vi "FilterDynamixelPositions.vi"(8 "Queue timeout (ms)":i32=8, 10 "DynamixelPosition Queue":refnum<queue>, 11 "NotifierReff":T1) -> ()   [LabVIEW 2013]
doc: "Performs and filtering that we want (default is no filtering) and writes the data to the notifier. If no data is in the queue this VI times out after 'Queue timeout (ms)' has passed and nothing is written to the notifier. When only one Dynamixel times, then '-1' is written to the timed out Dynamixel and the other torque is written to the notifier.\n\nEric Schneider, March 2014"
uses:
  Data/TypeDefs/Notifiers.ctl
  Data/TypeDefs/UTM Location.ctl
  Data/TypeDefs/Sail Set Suggestions.ctl
  Data/TypeDefs/Rudder Set Suggestions.ctl
  Data/TypeDefs/OverrideInformation.ctl
  Data/TypeDefs/OverrideMode.ctl
  Data/TypeDefs/MotorSetup.ctl
  Data/TypeDefs/DynamixelSetupInfo.ctl
  Data/TypeDefs/AirmarStatus.ctl
  Data/TypeDefs/HardwareOnline.ctl
panel:
  out "Old Rudder position":dbl
  out "New Rudder position":dbl
  out "New Jib position":dbl
  out "Old Jib position":dbl
  out "Old Main position":dbl
  out "New Main position":dbl
  out "Change for Rudder":i32
  out "Change for Jib":i32
  out "Change for Main":i32
  # "For Debugging"
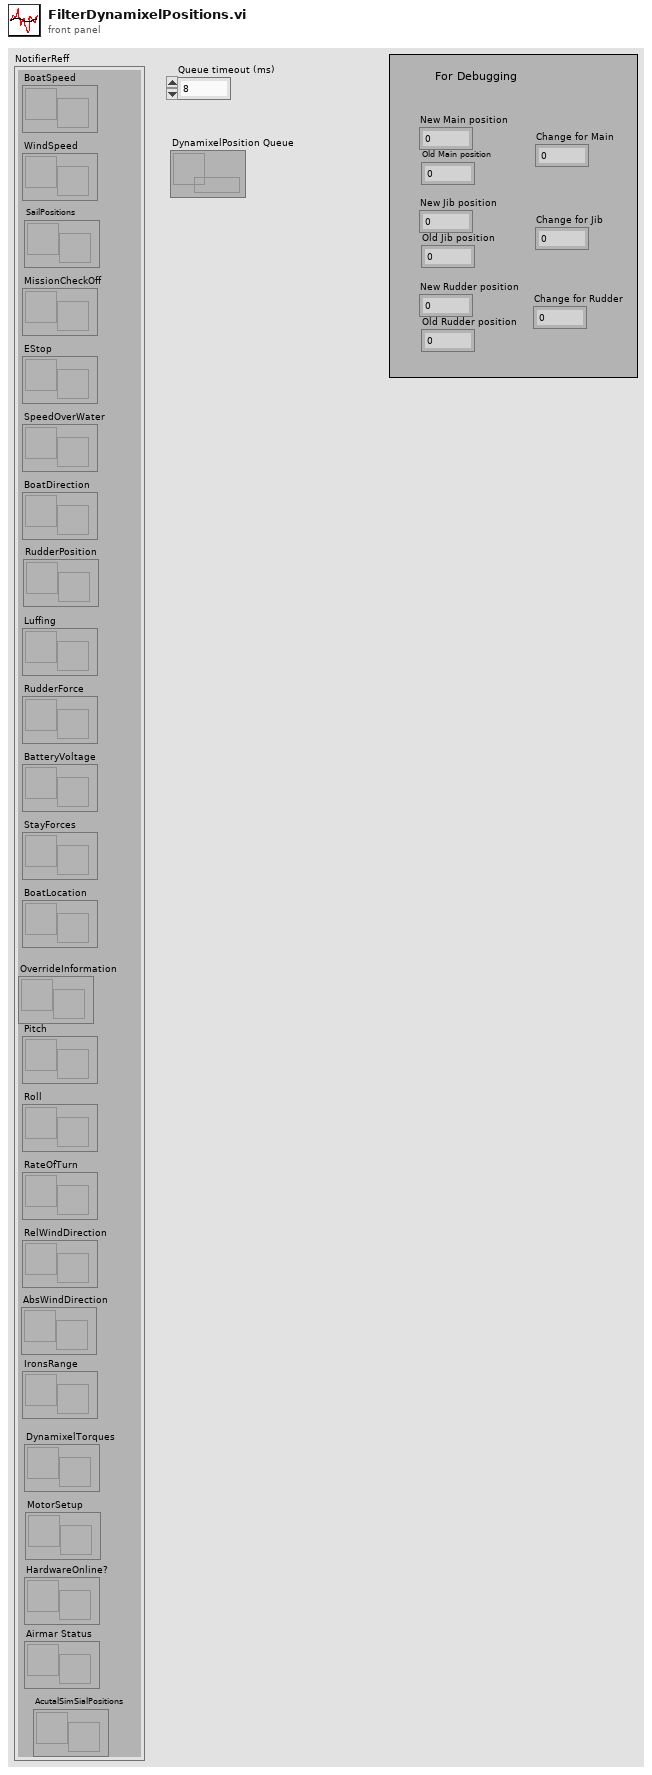
[diagram p1: front panel]
types:
  T1 = typedef "Notifiers.ctl" = cluster{"BoatSpeed":refnum<notifier>, "WindSpeed":refnum<notifier>, "MissionCheckOff":refnum<notifier>, "EStop":refnum<notifier>, "SpeedOverWater":refnum<notifier>, "BoatDirection":refnum<notifier>, "Luffing":refnum<notifier>, "RudderForce":refnum<notifier>, "BatteryVoltage":refnum<notifier>, "StayForces":refnum<notifier>, "BoatLocation":refnum<notifier>, "Pitch":refnum<notifier>, "Roll":refnum<notifier>, "RateOfTurn":refnum<notifier>, "RelWindDirection":refnum<notifier>, "SailPositions":refnum<notifier>, "RudderPosition":refnum<notifier>, "IronsRange":refnum<notifier>, "AbsWindDirection":refnum<notifier>, "OverrideInformation":refnum<notifier>, "DynamixelTorques":refnum<notifier>, "MotorSetup":refnum<notifier>, "Airmar Status":refnum<notifier>, "HardwareOnline?":refnum<notifier>, "AcutalSimSialPositions":refnum<notifier>}
  T2 = typedef "MotorSetup.ctl" = cluster{"Main Dynamixel Set Data":T3, "Rudder Dynamixel Set Data":T3, "Jib Dynamixel Set Data":T3}
  T3 = typedef "DynamixelSetupInfo.ctl" = cluster{"Lower Winch Bound":dbl, "Upper Winch Bound":dbl, "Reverse Winch Direction?":bool, "Dynamixel Cycle Number":i32}
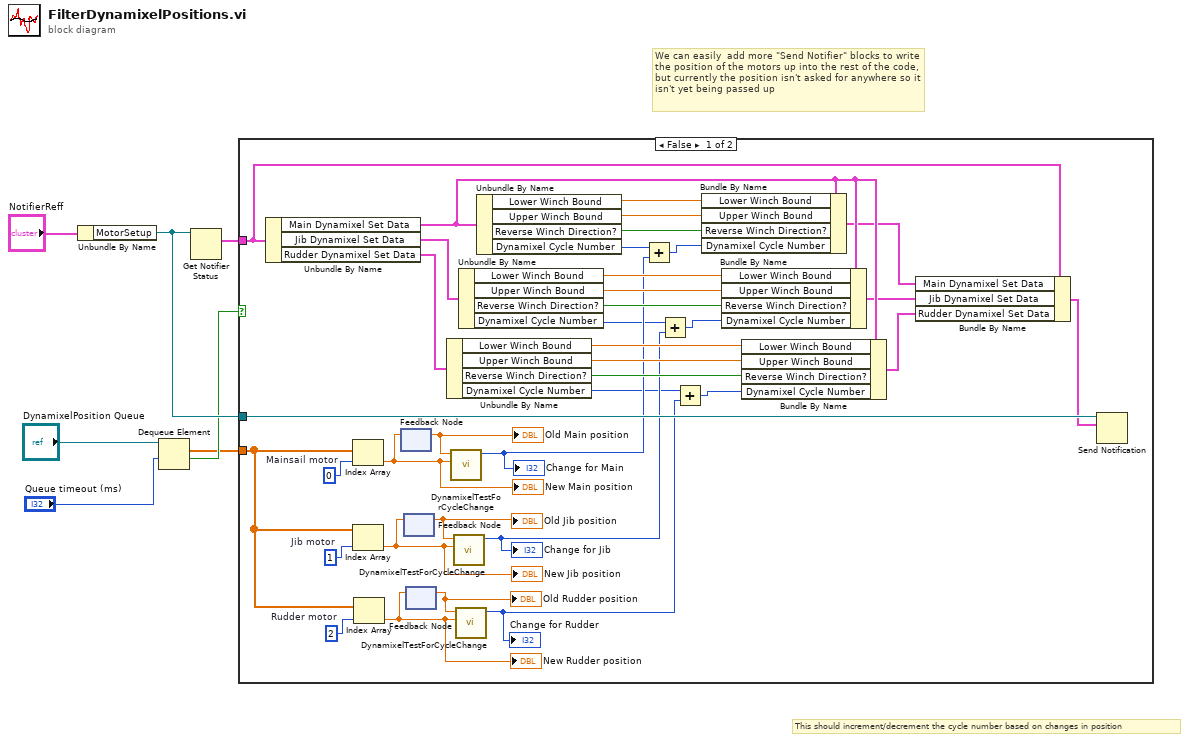
[diagram p0: block diagram]
diagram:
  # "We can easily  add more \"Send Notifier\" blocks to write the position of the motors up into the rest of the code, but currently the position isn't asked for anywhere so it isn't yet being passed up"
  # "This should increment/decrement the cycle number based on changes in position"
  n1 = Unbundle By Name("NotifierReff") -> ("MotorSetup"=w4:refnum<notifier>)
  n2 = Dequeue Element(queue="DynamixelPosition Queue", timeout in ms (-1)="Queue timeout (ms)") -> (element=w1:dbl[], timed out?=w2:bool)  [unwired: 1 in, 2 out]
  n3 = Get Notifier Status(notifier=w4) -> (current notification=w3:T2)  [unwired: 1 in, 4 out]
  n4 = case shown="False" w2 {
    tunnel: w4 -> [w42 _]
    tunnel: w3 -> [w37 _]
    tunnel: w1 -> [w23 _]
    frame False {
      w24 = 0  # Mainsail motor
      w25 = 1  # Jib motor
      w26 = 2  # Rudder motor
      n5 = Unbundle By Name(w37) -> ("Main Dynamixel Set Data"=w38:T3, "Jib Dynamixel Set Data"=w44:T3, "Rudder Dynamixel Set Data"=w43:T3)
      n6 = Index Array(array=w23, index=w24) -> (element=w22:dbl)
      "New Main position" <- w22
      n7 = Index Array(array=w23, index=w25) -> (element=w19:dbl)
      "New Jib position" <- w19
      n8 = Index Array(array=w23, index=w26) -> (element=w17:dbl)
      "New Rudder position" <- w17
      n9 = feedback #1() -> (w21:dbl)  [unwired: 1 in]
      "Old Main position" <- w21
      n10 = feedback-in #1(w22) -> ()
      n11 = feedback #2() -> (w20:dbl)  [unwired: 1 in]
      "Old Jib position" <- w20
      n12 = feedback-in #2(w19) -> ()
      n13 = feedback #3() -> (w18:dbl)  [unwired: 1 in]
      "Old Rudder position" <- w18
      n14 = feedback-in #3(w17) -> ()
      n15 = Unbundle By Name(w43) -> ("Lower Winch Bound"=w30:dbl, "Upper Winch Bound"=w29:dbl, "Reverse Winch Direction?"=w28:bool, "Dynamixel Cycle Number"=w10:i32)
      n16 = call "DynamixelTestForCycleChange.vi"("New position (deg)"=w22, "Old position (deg)"=w21) -> ("Dynamixel Cycle Number"=w15:i32)  [unwired: 9 in]
      "Change for Main" <- w15
      n17 = call "DynamixelTestForCycleChange.vi"("New position (deg)"=w19, "Old position (deg)"=w20) -> ("Dynamixel Cycle Number"=w12:i32)  [unwired: 9 in]
      "Change for Jib" <- w12
      n18 = call "DynamixelTestForCycleChange.vi"("New position (deg)"=w17, "Old position (deg)"=w18) -> ("Dynamixel Cycle Number"=w8:i32)  [unwired: 9 in]
      "Change for Rudder" <- w8
      n19 = Unbundle By Name(w44) -> ("Lower Winch Bound"=w33:dbl, "Upper Winch Bound"=w32:dbl, "Reverse Winch Direction?"=w31:bool, "Dynamixel Cycle Number"=w13:i32)
      n20 = Unbundle By Name(w38) -> ("Lower Winch Bound"=w39:dbl, "Upper Winch Bound"=w40:dbl, "Reverse Winch Direction?"=w41:bool, "Dynamixel Cycle Number"=w16:i32)
      n21 = Add(x=w16, y=w15) -> (x+y=w14:i32)
      n22 = Add(x=w13, y=w12) -> (x+y=w11:i32)
      n23 = Add(x=w10, y=w8) -> (x+y=w9:i32)
      n24 = Bundle By Name(cluster=w38, "Lower Winch Bound"=w39, "Upper Winch Bound"=w40, "Reverse Winch Direction?"=w41, "Dynamixel Cycle Number"=w14) -> (w36:T3)
      n25 = Bundle By Name(cluster=w38, "Lower Winch Bound"=w33, "Upper Winch Bound"=w32, "Reverse Winch Direction?"=w31, "Dynamixel Cycle Number"=w11) -> (w35:T3)
      n26 = Bundle By Name(cluster=w38, "Lower Winch Bound"=w30, "Upper Winch Bound"=w29, "Reverse Winch Direction?"=w28, "Dynamixel Cycle Number"=w9) -> (w34:T3)
      n27 = Bundle By Name(cluster=w37, "Main Dynamixel Set Data"=w36, "Jib Dynamixel Set Data"=w35, "Rudder Dynamixel Set Data"=w34) -> (w27:T2)
      n28 = Send Notification(notification=w27, notifier=w42) -> ()  [unwired: 1 in, 2 out]
    }
    frame True {
    }
  }
